vi "decodificator.vi"   [LabVIEW 2019]
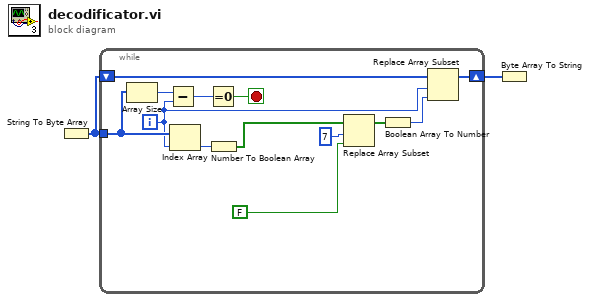
[diagram p0: block diagram]
diagram:
  n1 = String To Byte Array() -> (unsigned byte array=w2:u8[])  [unwired: 1 in]
  n2 = while {
    tunnel: w2 -> [w15]
    shift-right: [w8] -> w1
    shift-left: w2 -> [w7]
    i -> [w6]
    stop <- w12 stop-if-true
    n3 = Array Size(array=w15) -> (size(s)=w14:i32)
    n4 = Subtract(x=w14, y=w6) -> (x-y=w13:i32)
    n5 = Index Array(array=w15, index=w6) -> (element=w10:u8)
    n6 = Equal To 0?(x=w13) -> (x = 0?=w12:bool)
    n7 = Number To Boolean Array(number=w10) -> (Boolean array=w4:bool[])
    n8 = Replace Array Subset(array=w4, new element=FALSE, index=7) -> (w9:bool[])
    n9 = Boolean Array To Number(Boolean array=w9) -> (number=w5:u32)
    n10 = Replace Array Subset(array=w7, new element=w5, index=w6) -> (w8:u8[])
  }
  n11 = Byte Array To String(unsigned byte array=w1) -> ()  [unwired: 1 out]
